vi "AutoPlayParser.vi"(0 "Auto Play":string) -> (1 "Drive Command Strings":string[](array[string]), 2 "Drive Parameter Strings":string[](array[string]), 3 "Manipulator Command Strings":string[](array[string]), 4 "Manipulator Parameter Strings":string[](array[string]))   [LabVIEW 2019]
doc: "This VI parses a FRC 4265 standard autonomous play into two parallel sequences of steps and parameter strings. On sequence commands the robot's drive base while the other sequence commands the robot manipulator subsytems."
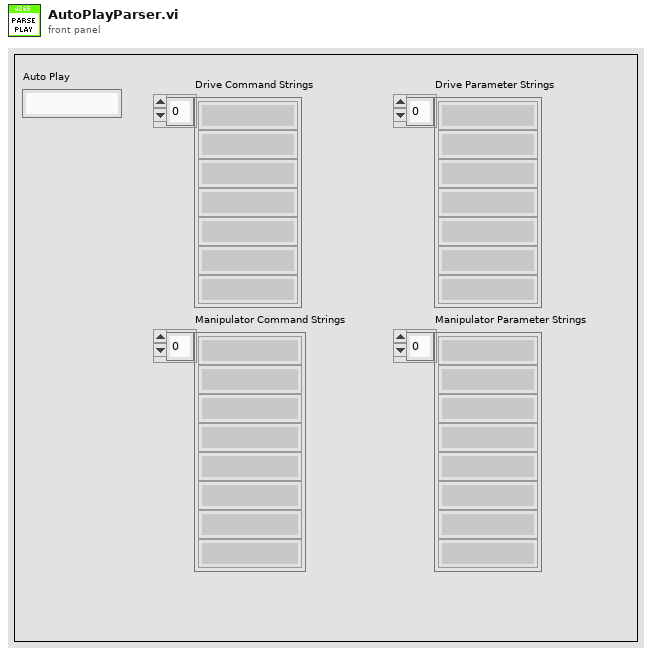
[diagram p1: front panel]
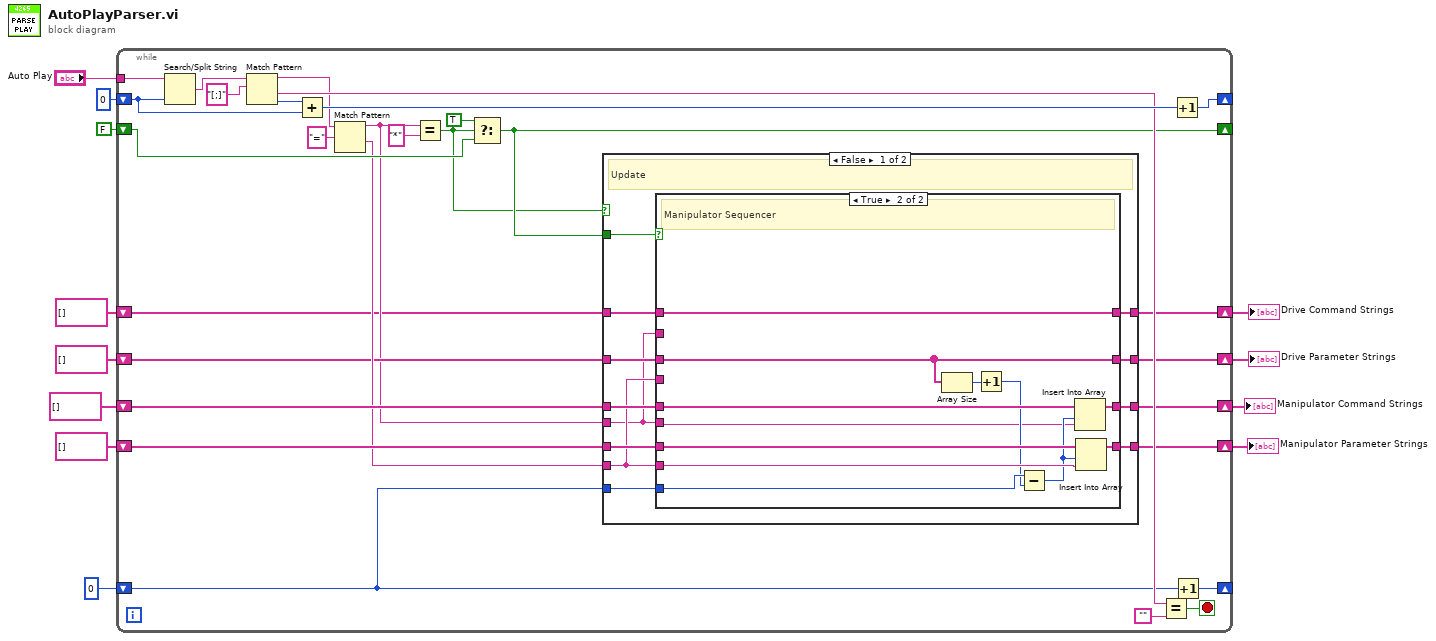
[diagram p0: block diagram]
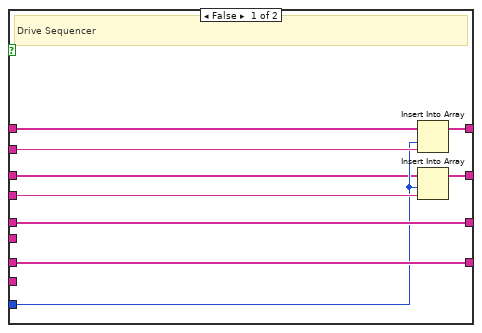
[diagram p2: hidden frame]
diagram:
  n1 = while {
    tunnel: "Auto Play" -> [w38]
    shift-right: [w33] -> _
    shift-left: 0 ("offset (0)") -> [w35]
    shift-right: [w29] -> _
    shift-left: 0 -> [w21]
    shift-right: [w28] -> w1
    shift-left: string[] [] -> [w27]
    shift-right: [w26] -> w10
    shift-left: string[] [] -> [w25]
    shift-right: [w20] -> _
    shift-left: FALSE -> [w22]
    shift-right: [w18] -> w8
    shift-left: string[] [] -> [w17]
    shift-right: [w15] -> w7
    shift-left: string[] [] -> [w14]
    stop <- w40 stop-if-true
    n2 = Search/Split String(string=w38, offset (0)=w35) -> (match + rest of string=w37:string)  [unwired: 1 in, 2 out]
    n3 = Match Pattern(string=w37, regular expression="[;]") -> (before substring=w30:string, after substring=w32:string, offset past match=w36:i32)  [unwired: 1 in, 1 out]
    n4 = Add(x=w36, y=w35) -> (x+y=w34:i32)
    n5 = Match Pattern(string=w30, regular expression="=") -> (before substring=w16:string, after substring=w19:string)  [unwired: 1 in, 2 out]
    n6 = Equal?(x=w16, y="*") -> (x = y?=w13:bool)
    n7 = Select(t=TRUE, s=w13, f=w22) -> (s? t:f=w20:bool)
    n8 = case shown="False" w13 {
      tunnel: [w53 w76] -> w28
      tunnel: w27 -> [w52 w76]
      tunnel: [w51 w75] -> w26
      tunnel: w25 -> [w50 w75]
      tunnel: w21 -> [w49 _]
      tunnel: w20 -> [w48 _]
      tunnel: w19 -> [w47 _]
      tunnel: [w46 w77] -> w18
      tunnel: w17 -> [w45 w77]
      tunnel: w16 -> [w44 _]
      tunnel: [w43 w78] -> w15
      tunnel: w14 -> [w42 w78]
      frame False {
        # "Update"
        n9 = case shown="True" w48 {
          tunnel: [w62 w74] -> w53
          tunnel: w52 -> [w62 w73]
          tunnel: w47 -> [_ w72]
          tunnel: [w61 w71] -> w51
          tunnel: w50 -> [w61 w70]
          tunnel: w44 -> [_ w63]
          tunnel: w49 -> [w55 w67]
          tunnel: w47 -> [w60 _]
          tunnel: [w59 w68] -> w46
          tunnel: w45 -> [w54 w68]
          tunnel: w44 -> [w58 _]
          tunnel: [w57 w69] -> w43
          tunnel: w42 -> [w56 w69]
          frame False {
            # "Drive Sequencer"
            n10 = Insert Into Array(array=w56, index=w55, new element=w58) -> (w57:string[])
            n11 = Insert Into Array(array=w54, index=w55, new element=w60) -> (w59:string[])
          }
          frame True {
            # "Manipulator Sequencer"
            n12 = Array Size(array=w68) -> (size(s)=w66:i32)
            n13 = Increment(x=w66) -> (x+1=w64:i32)
            n14 = Subtract(x=w67, y=w64) -> (x-y=w65:i32)
            n15 = Insert Into Array(array=w73, index=w65, new element=w63) -> (w74:string[])
            n16 = Insert Into Array(array=w70, index=w65, new element=w72) -> (w71:string[])
          }
        }
      }
      frame True {
        # "Skip Break Line"
      }
    }
    n17 = Equal?(x=w32, y="") -> (x = y?=w40:bool)
    n18 = Increment(x=w34) -> (x+1=w33:i32)
    n19 = Increment(x=w21) -> (x+1=w29:i32)
  }
  "Manipulator Parameter Strings" <- w10
  "Drive Parameter Strings" <- w8
  "Drive Command Strings" <- w7
  "Manipulator Command Strings" <- w1
